vi "FT_Search All.vi"(8 "error in (no error)":errorcluster, 11 "CTA Test#":string="CTA013A") -> (0 "error Out":errorcluster, 2 "All FT":T1(array[cluster]), 3 "Select Ft":T2)   [LabVIEW 2009]
uses:
  FT_Search all (state machine).ctl
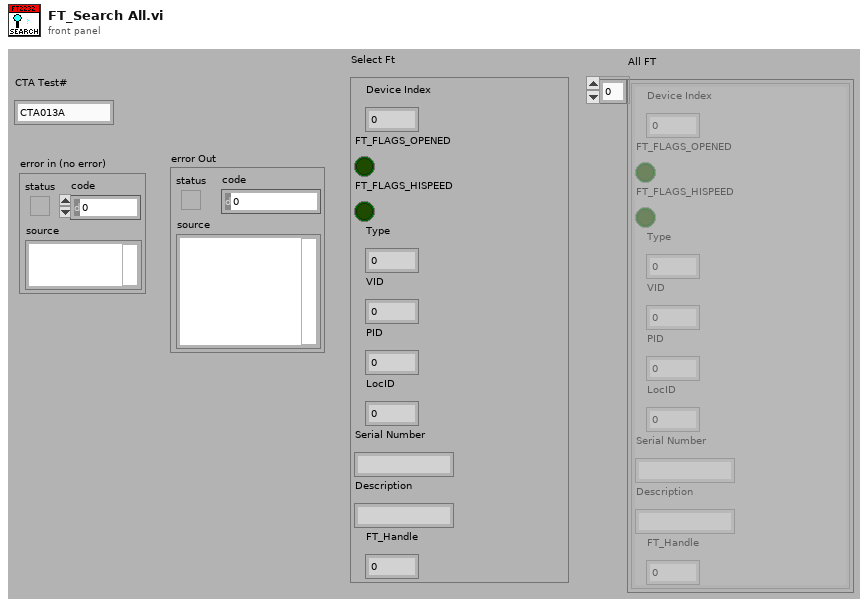
[diagram p1: front panel]
types:
  T1 = cluster{"Device Index":u32, "FT_FLAGS_OPENED":bool, "FT_FLAGS_HISPEED":bool, "Type":u32, "VID":u32, "PID":u32, "LocID":i32, "Serial Number":string, "Description":string, "FT_Handle":u32}[]
  T2 = cluster{"Device Index":u32, "FT_FLAGS_OPENED":bool, "FT_FLAGS_HISPEED":bool, "Type":u32, "VID":u32, "PID":u32, "LocID":i32, "Serial Number":string, "Description":string, "FT_Handle":u32}
  T3 = typedef "FT_Search all (state machine).ctl" = enum16{"Init", "Re_scan", "Close if Open", "Open FT", "Report FT", "Exit", "Error"}
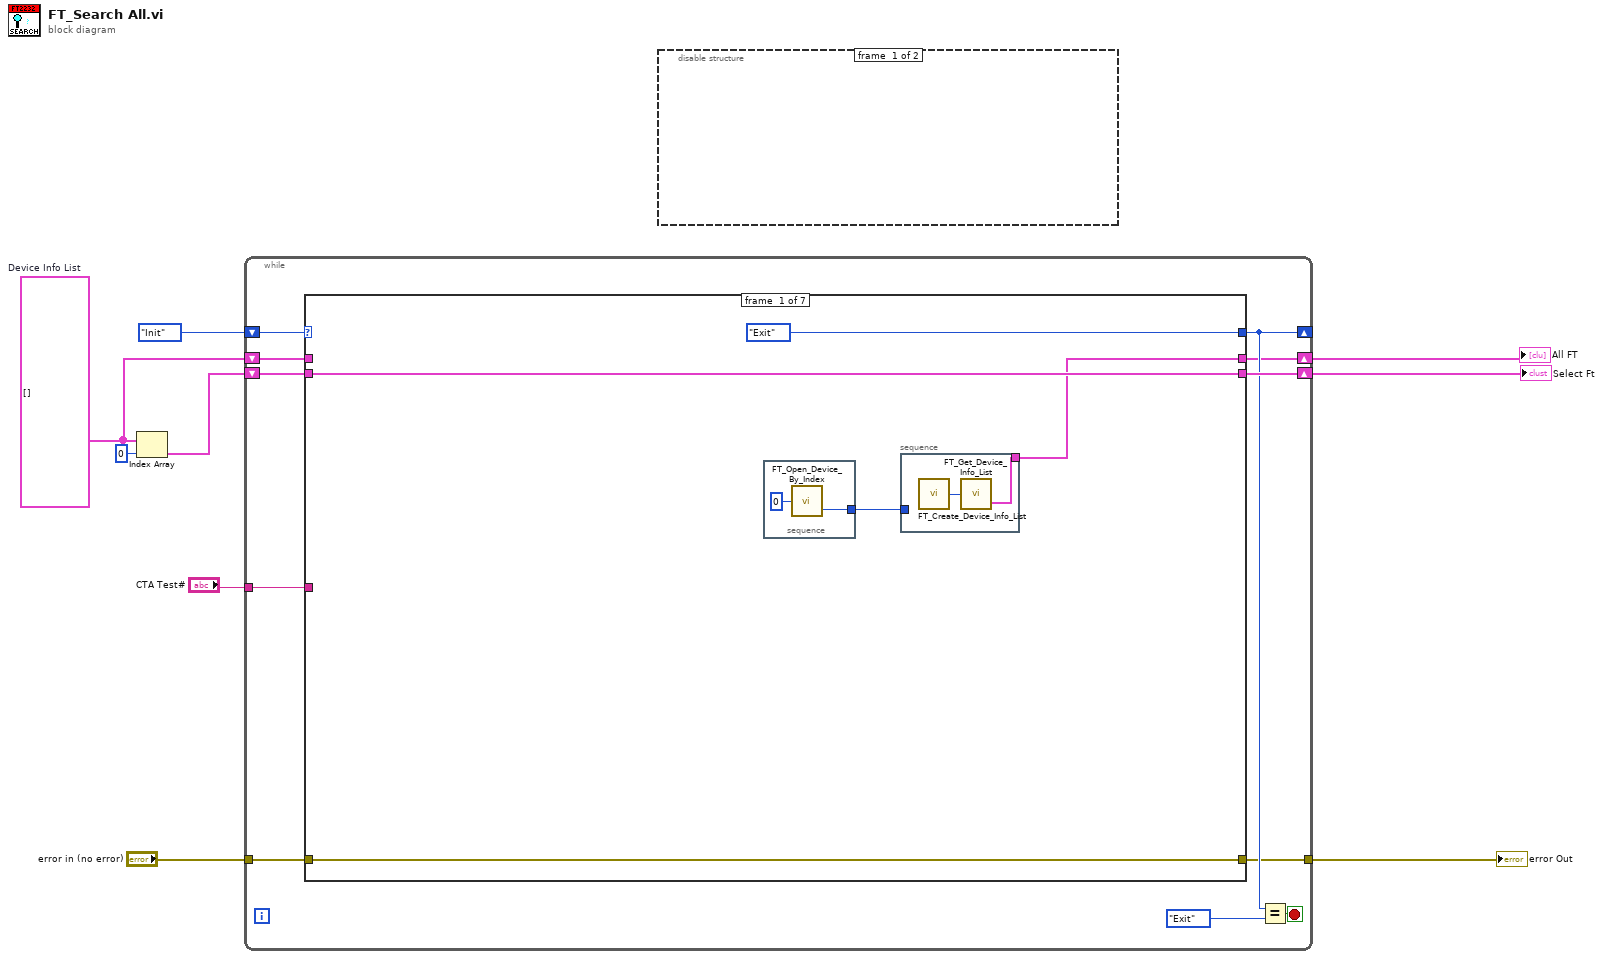
[diagram p0: block diagram]
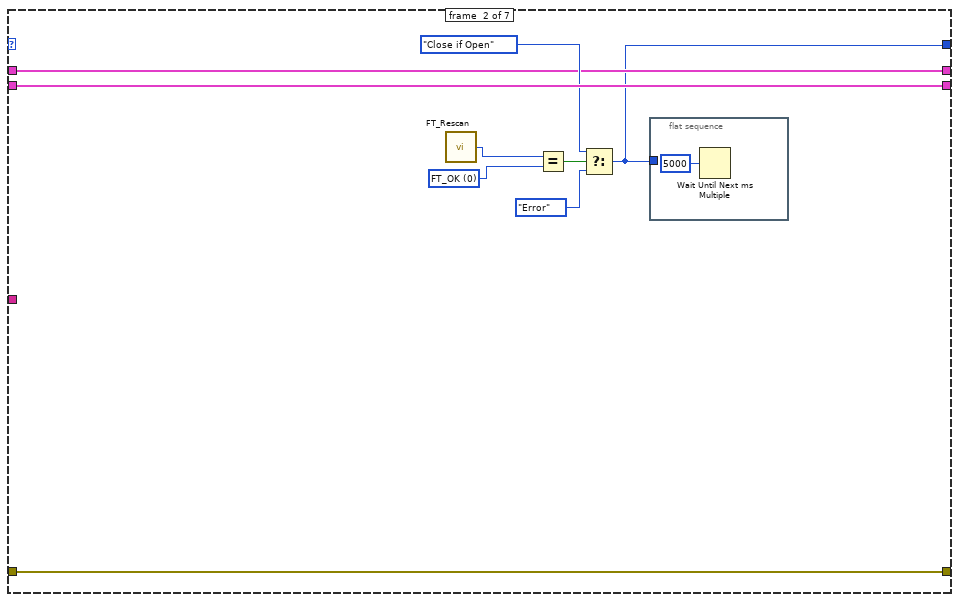
[diagram p3: hidden frame]
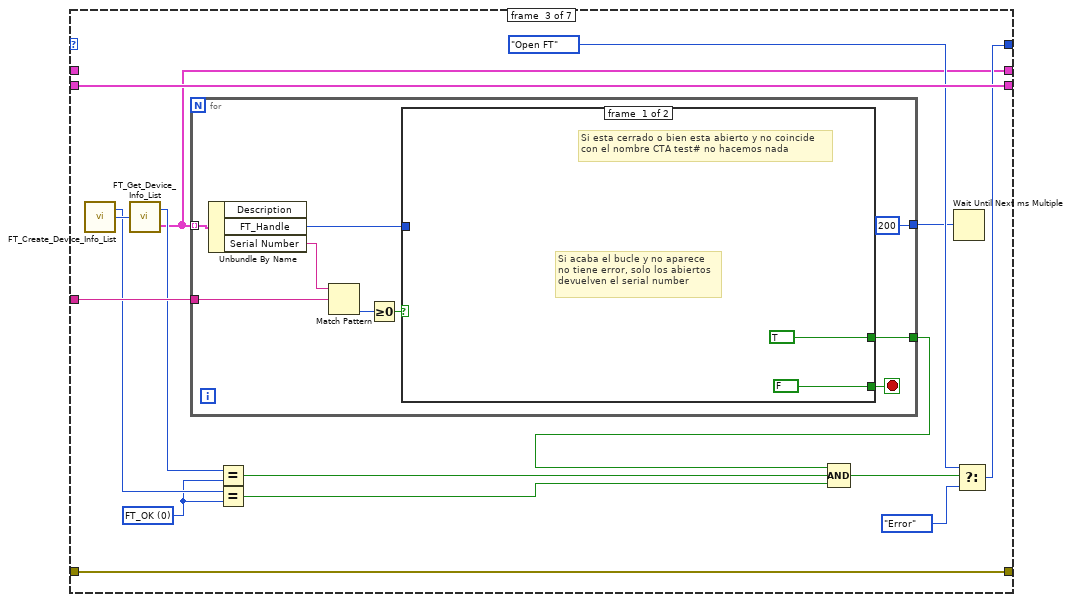
[diagram p4: hidden frame]
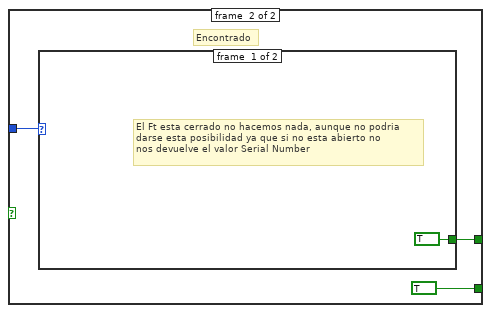
[diagram p5: hidden frame]
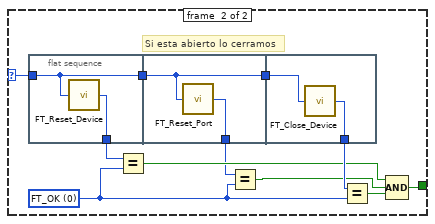
[diagram p6: hidden frame]
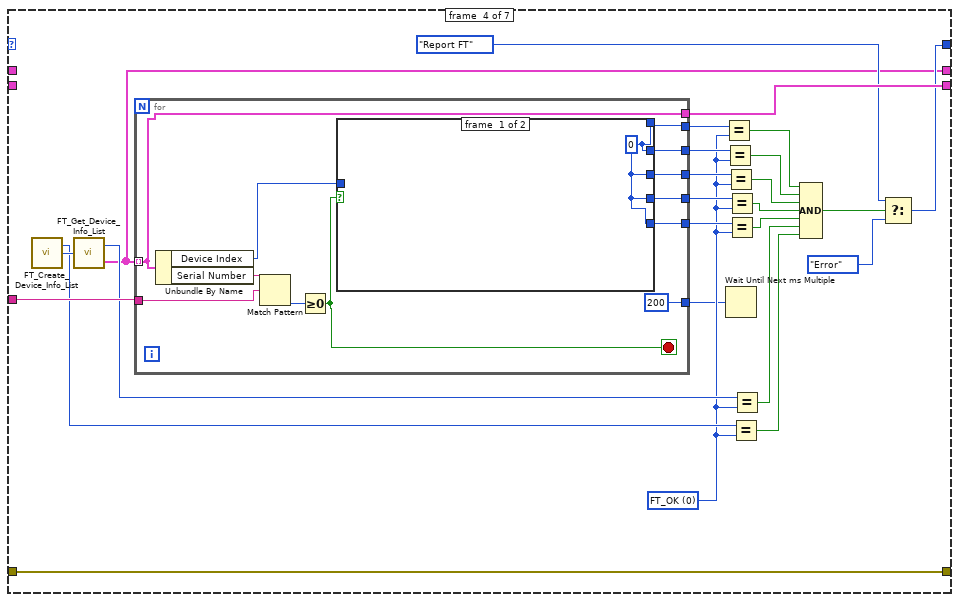
[diagram p7: hidden frame]
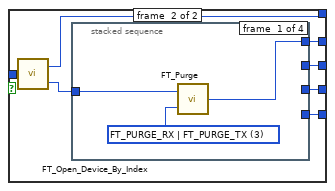
[diagram p8: hidden frame]
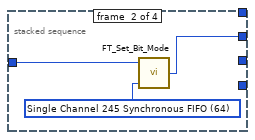
[diagram p9: hidden frame]
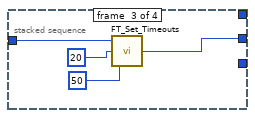
[diagram p10: hidden frame]
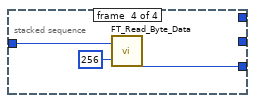
[diagram p11: hidden frame]
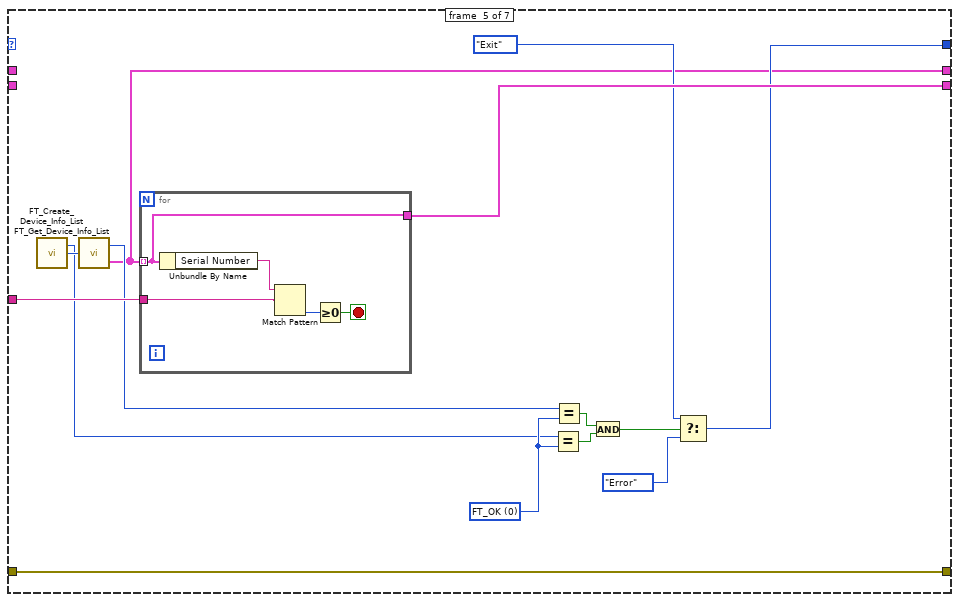
[diagram p12: hidden frame]
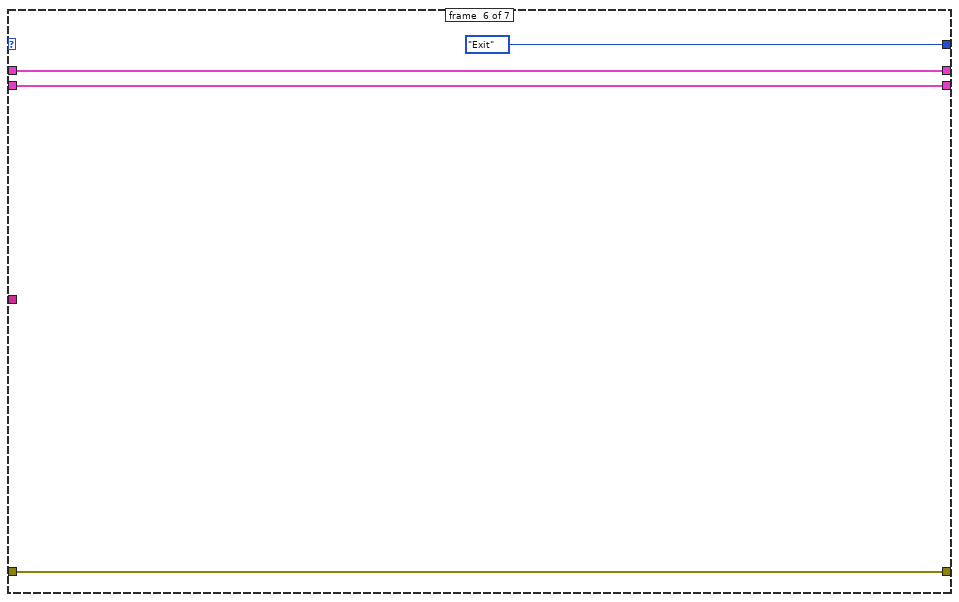
[diagram p13: hidden frame]
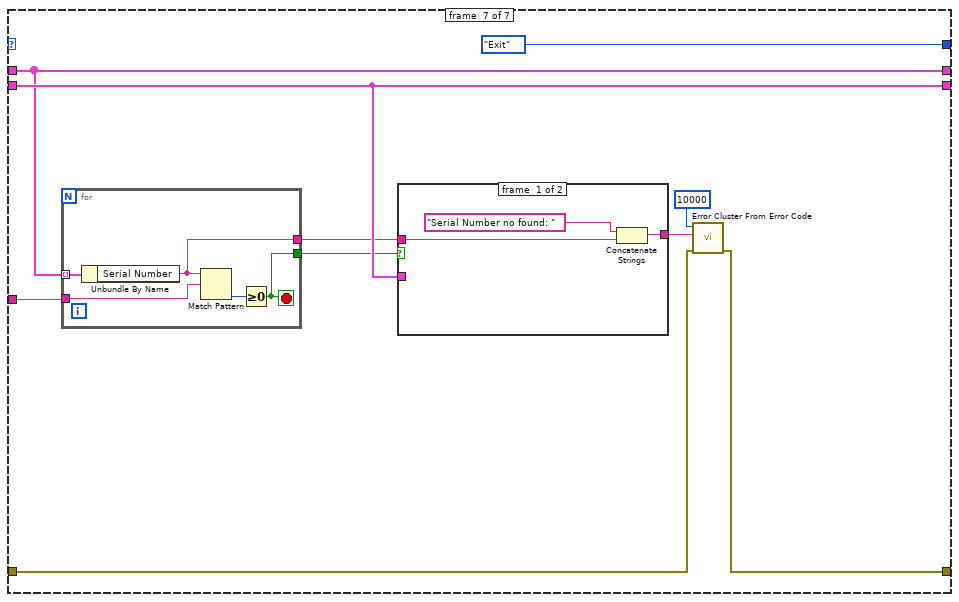
[diagram p14: hidden frame]
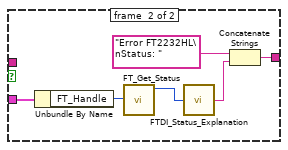
[diagram p15: hidden frame]
diagram:
  w3 = T1 []  # Device Info List
  n1 = Index Array(array=w3, index=0) -> (element=w6:T2)
  n2 = while {
    shift-right: [w15] -> _
    shift-left: FT_Search_all_(state_machine)."Init" ("State Search FT") -> [w20]
    tunnel: "CTA Test#" -> [w19]
    shift-right: [w16] -> w5
    shift-left: w6 -> [w18]
    tunnel: "error in (no error)" -> [w17]
    tunnel: [w12] -> w4
    shift-right: [w11] -> w2
    shift-left: w3 -> [w10]
    stop <- w13 stop-if-true
    n3 = case shown="\"Init\", Default" w20 {
      tunnel: w19 -> [_ _ w54 w111 w158 _ w171]
      tunnel: w18 -> [w25 w38 w53 _ _ w168 w177]
      tunnel: w17 -> [w23 w37 w52 w109 w156 w166 w174]
      tunnel: [w25 w38 w53 w110 w157 w168 w177] -> w16
      tunnel: [FT_Search_all_(state_machine)."Exit" ("State Search FT") w30 w42 w90 w147 FT_Search_all_(state_machine)."Exit" ("State Search FT") FT_Search_all_(state_machine)."Exit" ("State Search FT")] -> w15
      tunnel: [w23 w37 w52 w109 w156 w166 w173] -> w12
      tunnel: [w22 w31 w41 w89 w146 w165 w172] -> w11
      tunnel: w10 -> [_ w31 _ _ _ w165 w172]
      frame #0 {
        n4 = stacked-sequence {
          tunnel: [w26] -> w21
          frame #0 {
            n5 = call "FT_Open_Device_By_Index.vi"("Device Index"=u32 0) -> ("Handle"=w26:u32)  [unwired: 1 out]
          }
        }
        n6 = stacked-sequence {
          tunnel: [w28] -> w22
          tunnel: w21 -> [_]
          frame #0 {
            n7 = call "FT_Create_Device_Info_List.vi"() -> ("Number of Devices"=w29:u32)  [unwired: 1 out]
            n8 = call "FT_Get_Device_Info_List.vi"("Number Of Devices"=w29) -> ("Device Info List"=w28:T1)  [unwired: 1 out]
          }
        }
      }
      frame #1 {
        w36 = u32 0 items=["FT_OK", "FT_INVALID_HANDLE", "FT_DEVICE_NOT_FOUND", "FT_DEVICE_NOT_OPENED", "FT_IO_ERROR", "FT_INSUFFICIENT_RESOURCES", "FT_INVALID_PARAMETER", "FT_INVALID_BAUD_RATE", "FT_DEVICE_NOT_OPENED_FOR_ERASE", "FT_DEVICE_NOT_OPENED_FOR_WRITE", "FT_FAILED_TO_WRITE_DEVICE", "FT_EEPROM_READ_FAILED", "FT_EEPROM_WRITE_FAILED", "FT_EEPROM_ERASE_FAILED", "FT_EEPROM_NOT_PRESENT", "FT_EEPROM_NOT_PROGRAMMED", "FT_INVALID_ARGS", "FT_NOT_SUPPORTED", "FT_OTHER_ERROR"] ("FT_Status")
        n9 = call "FT_Rescan.vi"() -> ("FT_Status"=w35:u32)  [unwired: 1 in]
        n10 = Equal?(x=w35, y=w36) -> (x = y?=w34:bool)
        n11 = Select(t=FT_Search_all_(state_machine)."Close if Open" ("State Search FT"), s=w34, f=FT_Search_all_(state_machine)."Error") -> (s? t:f=w30:T3)
        n12 = flat-sequence {
          tunnel: w30 -> [_]
          frame #0 {
            n13 = Wait Until Next ms Multiple(millisecond multiple=u32 5000) -> ()  [unwired: 1 out]
          }
        }
      }
      frame #2 {
        w48 = u32 0 items=["FT_OK", "FT_INVALID_HANDLE", "FT_DEVICE_NOT_FOUND", "FT_DEVICE_NOT_OPENED", "FT_IO_ERROR", "FT_INSUFFICIENT_RESOURCES", "FT_INVALID_PARAMETER", "FT_INVALID_BAUD_RATE", "FT_DEVICE_NOT_OPENED_FOR_ERASE", "FT_DEVICE_NOT_OPENED_FOR_WRITE", "FT_FAILED_TO_WRITE_DEVICE", "FT_EEPROM_READ_FAILED", "FT_EEPROM_WRITE_FAILED", "FT_EEPROM_ERASE_FAILED", "FT_EEPROM_NOT_PRESENT", "FT_EEPROM_NOT_PROGRAMMED", "FT_INVALID_ARGS", "FT_NOT_SUPPORTED", "FT_OTHER_ERROR"] ("FT_Status")
        n14 = call "FT_Create_Device_Info_List.vi"() -> ("Number of Devices"=w55:u32, "FT_Status"=w50:u32)
        n15 = call "FT_Get_Device_Info_List.vi"("Number Of Devices"=w55) -> ("FT_Status"=w49:u32, "Device Info List"=w41:T1)
        n16 = for {
          tunnel: w41 -> [w62] mode=indexing
          tunnel: w54 -> [w60]
          tunnel: [w57] -> w47
          tunnel: [u32 200 ("millisecond multiple")] -> w40
          stop <- w63 stop-if-true
          n17 = Unbundle By Name(w62) -> ("FT_Handle"=w64:u32, "Serial Number"=w61:string)  [unwired: 1 out]
          n18 = Match Pattern(string=w61, regular expression=w60) -> (offset past match=w59:i32)  [unwired: 4 out]
          n19 = Greater Or Equal To 0?(x=w59) -> (x >= 0?=w58:bool)
          n20 = case shown="False" w58 {
            tunnel: w64 -> [_ w68]
            tunnel: [FALSE TRUE] -> w63
            tunnel: [TRUE w67] -> w57
            frame #0 {
              # "Si acaba el bucle y no aparece\nno tiene error, solo los abiertos\ndevuelven el serial number"
              # "Si esta cerrado o bien esta abierto y no coincide\ncon el nombre CTA test# no hacemos nada"
            }
            frame #1 {
              # "Encontrado"
              n21 = case shown="1, Default" w68 {
                selector: w68 -> [_ w71]
                tunnel: [TRUE w81] -> w67
                frame #0 {
                  # "El Ft esta cerrado no hacemos nada, aunque no podria\ndarse esta posibilidad ya que si no esta abierto no\nnos devuelve el valor Serial Number"
                }
                frame #1 {
                  w73 = u32 0 items=["FT_OK", "FT_INVALID_HANDLE", "FT_DEVICE_NOT_FOUND", "FT_DEVICE_NOT_OPENED", "FT_IO_ERROR", "FT_INSUFFICIENT_RESOURCES", "FT_INVALID_PARAMETER", "FT_INVALID_BAUD_RATE", "FT_DEVICE_NOT_OPENED_FOR_ERASE", "FT_DEVICE_NOT_OPENED_FOR_WRITE", "FT_FAILED_TO_WRITE_DEVICE", "FT_EEPROM_READ_FAILED", "FT_EEPROM_WRITE_FAILED", "FT_EEPROM_ERASE_FAILED", "FT_EEPROM_NOT_PRESENT", "FT_EEPROM_NOT_PROGRAMMED", "FT_INVALID_ARGS", "FT_NOT_SUPPORTED", "FT_OTHER_ERROR"] ("FT_Status")
                  # "Si esta abierto lo cerramos"
                  n22 = flat-sequence {
                    tunnel: w71 -> [w83]
                    tunnel: [w83] -> w80
                    tunnel: [w82] -> w72
                    tunnel: w80 -> [w85]
                    tunnel: [w85] -> w79
                    tunnel: [w84] -> w74
                    tunnel: w79 -> [w87]
                    tunnel: [w86] -> w78
                    frame #0 {
                      n23 = call "FT_Reset_Device.vi"("Handle"=w83) -> ("FT_Status"=w82:u32)
                    }
                    frame #1 {
                      n24 = call "FT_Reset_Port.vi"("Handle"=w85) -> ("FT_Status"=w84:u32)
                    }
                    frame #2 {
                      n25 = call "FT_Close_Device.vi"("Handle"=w87) -> ("FT_Status"=w86:u32)
                    }
                  }
                  n26 = Equal?(x=w72, y=w73) -> (x = y?=w75:bool)
                  n27 = Equal?(x=w74, y=w73) -> (x = y?=w76:bool)
                  n28 = Equal?(x=w78, y=w73) -> (x = y?=w77:bool)
                  n29 = Compound Arithmetic op=AND(w75, w76, w77) -> (w81:bool)
                }
              }
            }
          }
        }
        n30 = Equal?(x=w49, y=w48) -> (x = y?=w46:bool)
        n31 = Equal?(x=w50, y=w48) -> (x = y?=w45:bool)
        n32 = Compound Arithmetic op=AND(w47, w46, w45) -> (w44:bool)
        n33 = Wait Until Next ms Multiple(millisecond multiple=w40) -> ()  [unwired: 1 out]
        n34 = Select(t=FT_Search_all_(state_machine)."Open FT" ("State Search FT"), s=w44, f=FT_Search_all_(state_machine)."Error") -> (s? t:f=w42:T3)
      }
      frame #3 {
        w101 = u32 0 items=["FT_OK", "FT_INVALID_HANDLE", "FT_DEVICE_NOT_FOUND", "FT_DEVICE_NOT_OPENED", "FT_IO_ERROR", "FT_INSUFFICIENT_RESOURCES", "FT_INVALID_PARAMETER", "FT_INVALID_BAUD_RATE", "FT_DEVICE_NOT_OPENED_FOR_ERASE", "FT_DEVICE_NOT_OPENED_FOR_WRITE", "FT_FAILED_TO_WRITE_DEVICE", "FT_EEPROM_READ_FAILED", "FT_EEPROM_WRITE_FAILED", "FT_EEPROM_ERASE_FAILED", "FT_EEPROM_NOT_PRESENT", "FT_EEPROM_NOT_PROGRAMMED", "FT_INVALID_ARGS", "FT_NOT_SUPPORTED", "FT_OTHER_ERROR"] ("FT_Status")
        n35 = call "FT_Create_Device_Info_List.vi"() -> ("Number of Devices"=w112:u32, "FT_Status"=w107:u32)
        n36 = call "FT_Get_Device_Info_List.vi"("Number Of Devices"=w112) -> ("FT_Status"=w108:u32, "Device Info List"=w89:T1)
        n37 = for {
          tunnel: w89 -> [w123] mode=indexing
          tunnel: w111 -> [w114]
          tunnel: [w123] -> w110
          tunnel: [w122] -> w106
          tunnel: [w121] -> w105
          tunnel: [w120] -> w104
          tunnel: [w119] -> w103
          tunnel: [w118] -> w102
          tunnel: [u32 200 ("millisecond multiple")] -> w88
          stop <- w113 stop-if-true
          n38 = Unbundle By Name(w123) -> ("Device Index"=w124:u32, "Serial Number"=w115:string)
          n39 = Match Pattern(string=w115, regular expression=w114) -> (offset past match=w116:i32)  [unwired: 4 out]
          n40 = Greater Or Equal To 0?(x=w116) -> (x >= 0?=w113:bool)
          n41 = case shown="True" w113 {
            tunnel: w124 -> [_ w132]
            tunnel: [w125 w130] -> w122
            tunnel: [w125 w129] -> w121
            tunnel: [w125 w128] -> w120
            tunnel: [w125 w127] -> w119
            tunnel: [w125 w126] -> w118
            frame #0 {
              w125 = u32 0 ("FT_Status")
            }
            frame #1 {
              n42 = call "FT_Open_Device_By_Index.vi"("Device Index"=w132) -> ("FT_Status"=w130:u32, "Handle"=w131:u32)
              n43 = stacked-sequence {
                tunnel: w131 -> [w135 w137 w140 w145]
                tunnel: [w133 _ _ _] -> w129
                tunnel: [_ w136 _ _] -> w128
                tunnel: [_ _ w139 _] -> w127
                tunnel: [_ _ _ w143] -> w126
                frame #0 {
                  w134 = u32 3 items=["FT_PURGE_RX"=1, "FT_PURGE_TX"=2, "FT_PURGE_RX | FT_PURGE_TX"=3] ("Purge Flags")
                  n44 = call "FT_Purge.vi"("Purge Flags"=w134, "Handle"=w135) -> ("FT_Status"=w133:u32)
                }
                frame #1 {
                  w138 = u8 64 items=["Reset Bit Mode"=0, "Asynchronous Bit Bang"=1, "MPSSE"=2, "Synchronous Bit Bang"=4, "MCU Host Bus Emulation"=8, "Fast Opto-Isolated Serial"=16, "CBUS Bit Bang"=32, "Single Channel 245 Synchronous FIFO"=64] ("Bit Mode")
                  n45 = call "FT_Set_Bit_Mode.vi"("Bit Mode"=w138, "Handle"=w137) -> ("FT_Status"=w136:u32)  [unwired: 1 in]
                }
                frame #2 {
                  n46 = call "FT_Set_Timeouts.vi"("Write Timeout"=u32 50, "Read Timeout"=u32 20, "Handle"=w140) -> ("FT_Status"=w139:u32)
                }
                frame #3 {
                  n47 = call "FT_Read_Byte_Data.vi"("Handle"=w145, "Bytes To Read"=u32 256) -> ("FT_Status"=w143:u32)  [unwired: 2 out]
                }
              }
            }
          }
        }
        n48 = Equal?(x=w106, y=w101) -> (x = y?=w100:bool)
        n49 = Equal?(x=w105, y=w101) -> (x = y?=w99:bool)
        n50 = Equal?(x=w104, y=w101) -> (x = y?=w98:bool)
        n51 = Wait Until Next ms Multiple(millisecond multiple=w88) -> ()  [unwired: 1 out]
        n52 = Equal?(x=w103, y=w101) -> (x = y?=w97:bool)
        n53 = Equal?(x=w102, y=w101) -> (x = y?=w96:bool)
        n54 = Equal?(x=w107, y=w101) -> (x = y?=w94:bool)
        n55 = Equal?(x=w108, y=w101) -> (x = y?=w95:bool)
        n56 = Compound Arithmetic op=AND(w100, w99, w98, w97, w96, w95, w94) -> (w92:bool)
        n57 = Select(t=FT_Search_all_(state_machine)."Report FT" ("State Search FT"), s=w92, f=FT_Search_all_(state_machine)."Error") -> (s? t:f=w90:T3)
      }
      frame #4 {
        w155 = u32 0 items=["FT_OK", "FT_INVALID_HANDLE", "FT_DEVICE_NOT_FOUND", "FT_DEVICE_NOT_OPENED", "FT_IO_ERROR", "FT_INSUFFICIENT_RESOURCES", "FT_INVALID_PARAMETER", "FT_INVALID_BAUD_RATE", "FT_DEVICE_NOT_OPENED_FOR_ERASE", "FT_DEVICE_NOT_OPENED_FOR_WRITE", "FT_FAILED_TO_WRITE_DEVICE", "FT_EEPROM_READ_FAILED", "FT_EEPROM_WRITE_FAILED", "FT_EEPROM_ERASE_FAILED", "FT_EEPROM_NOT_PRESENT", "FT_EEPROM_NOT_PROGRAMMED", "FT_INVALID_ARGS", "FT_NOT_SUPPORTED", "FT_OTHER_ERROR"] ("FT_Status")
        n58 = call "FT_Create_Device_Info_List.vi"() -> ("Number of Devices"=w159:u32, "FT_Status"=w154:u32)
        n59 = call "FT_Get_Device_Info_List.vi"("Number Of Devices"=w159) -> ("FT_Status"=w153:u32, "Device Info List"=w146:T1)
        n60 = for {
          tunnel: w146 -> [w160] mode=indexing
          tunnel: w158 -> [w162]
          tunnel: [w160] -> w157
          stop <- w161 stop-if-true
          n61 = Unbundle By Name(w160) -> ("Serial Number"=w163:string)
          n62 = Match Pattern(string=w163, regular expression=w162) -> (offset past match=w164:i32)  [unwired: 4 out]
          n63 = Greater Or Equal To 0?(x=w164) -> (x >= 0?=w161:bool)
        }
        n64 = Equal?(x=w154, y=w155) -> (x = y?=w151:bool)
        n65 = Equal?(x=w153, y=w155) -> (x = y?=w152:bool)
        n66 = And(x=w152, y=w151) -> (x .and. y?=w149:bool)
        n67 = Select(t=FT_Search_all_(state_machine)."Exit" ("State Search FT"), s=w149, f=FT_Search_all_(state_machine)."Error") -> (s? t:f=w147:T3)
      }
      frame #5 {
      }
      frame #6 {
        n68 = for {
          tunnel: w172 -> [w191] mode=indexing
          tunnel: w171 -> [w190]
          tunnel: [w189] -> w170
          tunnel: [w188] -> w169
          stop <- w189 stop-if-true
          n69 = Unbundle By Name(w191) -> ("Serial Number"=w188:string)
          n70 = Match Pattern(string=w188, regular expression=w190) -> (offset past match=w192:i32)  [unwired: 4 out]
          n71 = Greater Or Equal To 0?(x=w192) -> (x >= 0?=w189:bool)
        }
        n72 = case shown="True" w170 {
          tunnel: w177 -> [_ w187]
          tunnel: [w181 w183] -> w175
          tunnel: w169 -> [w179 _]
          frame #0 {
            n73 = Concatenate Strings("Serial Number no found: ", w179) -> (w181:string)
          }
          frame #1 {
            n74 = Unbundle By Name(w187) -> ("FT_Handle"=w186:u32)
            n75 = call "FT_Get_Status.vi"("Handle"=w186) -> ("FT_Status"=w184:u32)  [unwired: 3 out]
            n76 = call "FTDI_Status_Explanation.vi"("FT_Status"=w184) -> ("Status String"=w182:string)
            n77 = Concatenate Strings("Error FT2232HL\nStatus: ", w182) -> (w183:string)
          }
        }
        n78 = call <vilib>:"Error Cluster From Error Code.vi"("error in (no error)"=w174, "error message (\"\")"=w175, "error code (0)"=10000 ("error code (no error:0)")) -> ("error out"=w173:errorcluster)  [unwired: 1 in, 5 out]
      }
    }
    n79 = Equal?(x=w15, y=FT_Search_all_(state_machine)."Exit" ("State Search FT")) -> (x = y?=w13:bool)
  }
  "Select Ft" <- w5
  "error Out" <- w4
  "All FT" <- w2
  n80 = disable-structure shown="Enabled" {
    frame #0 {
    }
    frame #1 {
    }
  }
